vi "GetTCPanel.vi"(6 "error in":errorcluster, 9 "ip":string="10.215.142.232") -> (0 "error out":errorcluster, 3 "panel":refnum<vi>)   [LabVIEW 2017]
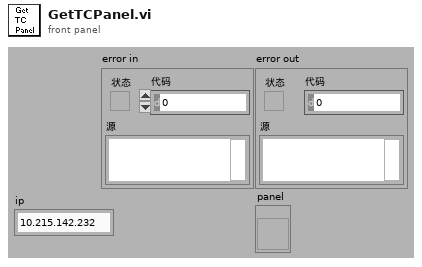
[diagram p1: front panel]
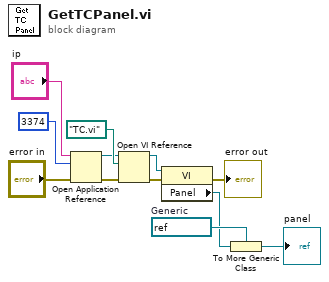
[diagram p0: block diagram]
diagram:
  w3 = refnum<vi> refnum  # Generic
  n1 = Open Application Reference(8:"error in", 10:u16 3374 ("端口号或服务名称(3363)"), 11:"ip") -> (0:w7:errorcluster, 3:w10:refnum<vi>)  [unwired: 1 out]
  n2 = Open VI Reference(application reference (local)=w10, vi path=path "TC.vi" ("VI路径"), error in (no error)=w7) -> (vi reference=w12:refnum<vi>, error out=w6:errorcluster)  [unwired: 3 out]
  n3 = property class="VI"(reference=w12, error in=w6) -> (error out=→"error out":errorcluster, "Panel"=w2:refnum<vi>)  [unwired: 1 out]
  n4 = To More Generic Class(target class=w3, reference=w2) -> (generic class reference=→"panel":refnum<vi>)
